vi "SVL Max-Min Level (N Ch).vi"(6 "restart averaging (F)":bool, 8 "error in (no error)":errorcluster, 11 "scaled signals [EU]":waveform(dbl)[](array[waveform])) -> (0 "error out":errorcluster, 2 "unit labels":string[](array[string]), 3 "max-min levels [EU]":dbl[](array[numeric]) format="%.2f", 5 "min levels [EU]":dbl[](array[numeric]) format="%.2f", 7 "max levels [EU]":dbl[](array[numeric]) format="%.2f")   [LabVIEW 2017, in "SoundVib_VibrationLevel.lvlib"]
doc: "Computes the maximum and minimum levels of all previous values and the difference between the maximum and minimum levels of <B>scaled signal [EU]</B> or <B>even-angle signal [EU]</B>. <B>scaled signal [EU]</B> should have a zero DC component. You can attenuate the DC component with hardware AC-coupling filters and with software high-pass filters. Wire data to the <B>scaled signal [EU]</B> input to determine the polymorphic instance to use or manually select the instance."
uses:
  <vilib>/addons/Sound and Vibration/svt_Level/SoundVib_VibrationLevel.lvlib
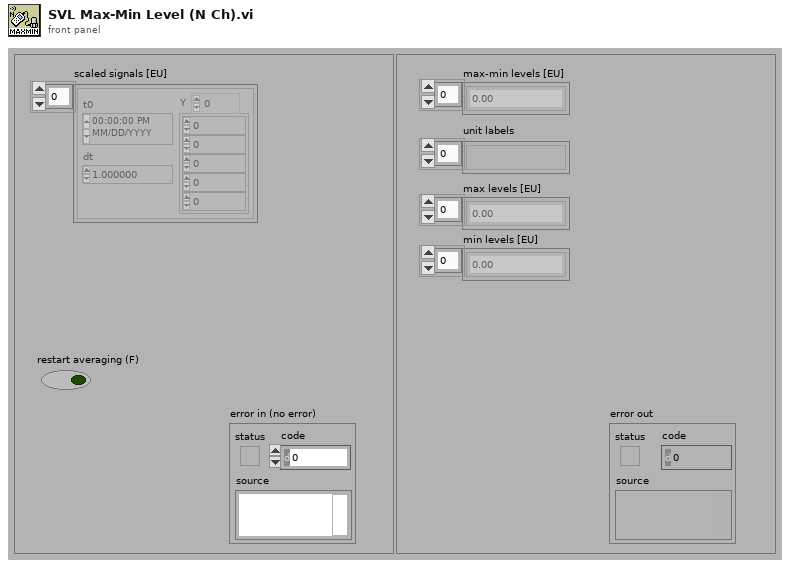
[diagram p1: front panel]
types:
  T1 = enum16{"RMS", "Running RMS", "Exp avg  ", "Dec exp avg ", "Peak", "Crest"}
  T2 = enum16{"Reset filter", "Restart averaging", "Continue processing"}
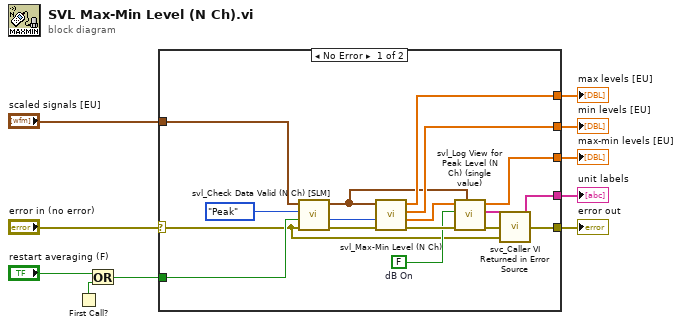
[diagram p0: block diagram]
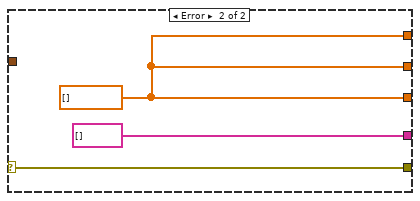
[diagram p2: hidden frame]
diagram:
  n1 = First Call?() -> (First Call?: T/F=w6:bool)
  n2 = Or(x="restart averaging (F)", y=w6) -> (x .or. y?=w4:bool)
  n3 = case shown="No Error" "error in (no error)" {
    selector: "error in (no error)" -> [w11 w29]
    tunnel: [w22 w29] -> w10
    tunnel: [w25 string[] [] ("unit label [ ]")] -> w9
    tunnel: [w24 w27] -> w8
    tunnel: "scaled signals [EU]" -> [w13 _]
    tunnel: w4 -> [w20 _]
    tunnel: [w18 w27] -> w2
    tunnel: [w17 w27] -> w1
    frame No Error {
      w14 = FALSE  # dB On
      n4 = call <vilib>:"svl_Check Data Valid (N Ch) [SLM].vi"("error in (no error)"=w11, "restart averaging (F)"=w20, "level analysis"=T1."Peak" ("Level Analysis"), "scaled signals [EU]"=w13) -> ("error out"=w21:errorcluster, "processing state"=w19:T2, "dup scaled signals [EU]"=w12:waveform(dbl)[])  [unwired: 5 in]
      n5 = call <vilib>:"svl_Max-Min Level (N Ch).vi"("error in (no error)"=w21, "processing state"=w19, "scaled signal(s)"=w12) -> ("error out"=w23:errorcluster, "max-min level(s)"=w15:dbl[], "min level(s)"=w17:dbl[], "max level(s)"=w18:dbl[])  [unwired: 5 in]
      n6 = call <vilib>:"svl_Log View for Peak Level (N Ch) (single value).vi"("scaled signals [EU]"=w12, "error in (no error)"=w23, "dB On (T)"=w14, "peak levels [EU]"=w15) -> ("error out"=w26:errorcluster, "unit label [ ]"=w25:string[], "peak levels [EU]"=w24:dbl[])  [unwired: 5 in]
      n7 = call <vilib>:"svc_Caller VI Returned in Error Source.vi"("warning input to caller"=w11, "error in (no error)"=w26) -> ("error out"=w22:errorcluster)  [unwired: 3 in]
    }
    frame Error {
      w27 = dbl[] [] ("energy levels [EU^2 rms]")
    }
  }
  "max-min levels [EU]" <- w8
  "unit labels" <- w9
  "error out" <- w10
  "max levels [EU]" <- w2
  "min levels [EU]" <- w1
